vi "Configure Frequency.vi"(5 "Sweep time (ms)":dbl caption="Sweep time for zero span (ms)", 7 "Mode (Center/Span)":enum16{"Center/Span", "Start/Stop"}(ring), 8 "error in (no error)":errorcluster, 9 "Span/Stop Frequency [Hz]":dbl, 10 "Center/Start Frequency [Hz]":dbl, 11 "MXA in":refnum<class "MXA.lvclass">) -> (0 "error out":errorcluster, 3 "MXA out":refnum<class "MXA.lvclass">)   [LabVIEW 2020, in "MXA.lvclass"]
uses:
  MXA.lvclass
  C:/Sandbox/Git_Sandbox/WiSpry Test Framework source code (LV20)/WiSpry Test Framework/Instruments/Instrument.lvclass
  C:/Sandbox/Git_Sandbox/WiSpry Test Framework source code (LV20)/WiSpry Test Framework/Instruments/Spectrum Analyzer/Spectrum Analyzer.lvclass
  Instrument.lvclass/Instrument.ctl
  Spectrum Analyzer.lvclass/Spectrum Analyzer.ctl
  <instrlib>/Agilent MXA Series/Public/Configure/Configure Frequency (Start Stop).vi
  <instrlib>/Agilent MXA Series/Public/Configure/Configure Frequency (Center Span).vi
  Instrument.lvclass
  <instrlib>/Agilent MXA Series/Agilent MXA Series.lvlib
  Spectrum Analyzer.lvclass
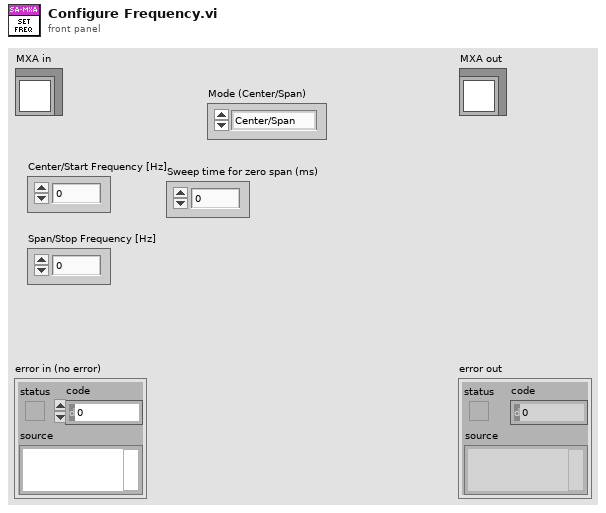
[diagram p1: front panel]
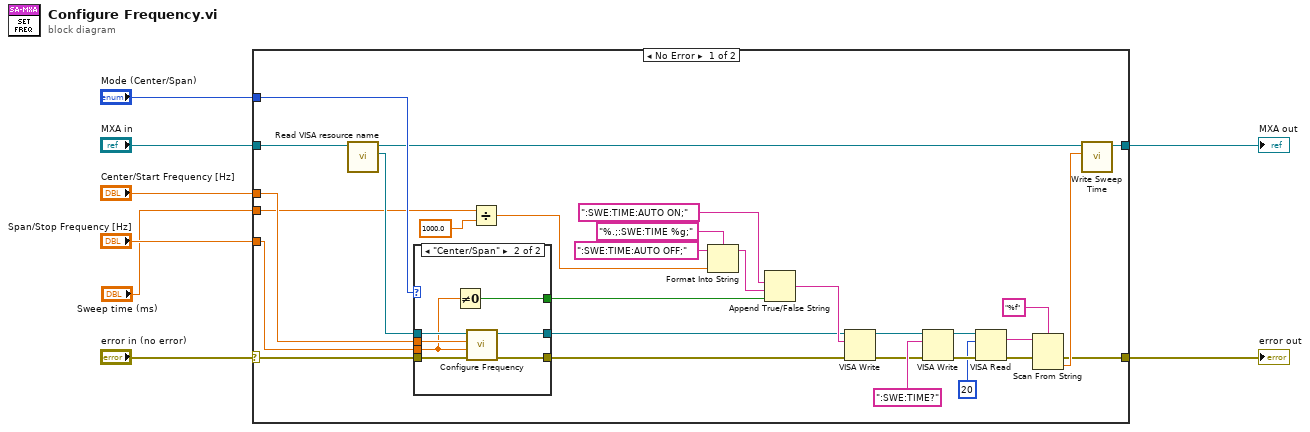
[diagram p0: block diagram]
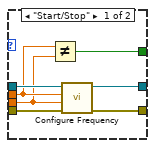
[diagram p2: hidden frame]
diagram:
  n1 = case shown="No Error" "error in (no error)" {
    selector: "error in (no error)" -> [w36 w54]
    tunnel: "MXA in" -> [w38 w53]
    tunnel: [w24 w54] -> w7
    tunnel: [w22 w53] -> w6
    tunnel: "Center/Start Frequency [Hz]" -> [w35 _]
    tunnel: "Span/Stop Frequency [Hz]" -> [w34 _]
    tunnel: "Mode (Center/Span)" -> [w33 _]
    tunnel: "Sweep time (ms)" -> [w16 _]
    frame No Error {
      n2 = call "Read VISA resource name.vi"("Instrument in"=w38) -> ("VISA resource name"=w37:refnum<visa-resource-name>, "Instrument out"=w23:refnum<class "MXA.lvclass">)  [unwired: 9 in]
      n3 = case shown="\"Center/Span\"" w33 {
        tunnel: w37 -> [w45 w52]
        tunnel: w36 -> [w44 w51]
        tunnel: [w43 w50] -> w11
        tunnel: w35 -> [w41 w49]
        tunnel: w34 -> [w40 w47]
        tunnel: [w42 w48] -> w12
        tunnel: [w39 w46] -> w17
        frame "Start/Stop" {
          n4 = Not Equal?(x=w41, y=w40) -> (x != y?=w39:bool)
          n5 = call-poly <instrlib>:"Configure Frequency.vi"("error in (no error)"=w44, "Stop Frequency (2.65E+10 Hz)"=w40, "Start Frequency (1E+7 Hz)"=w41, "VISA resource name"=w45) -> ("error out"=w43:errorcluster, "VISA resource name out"=w42:refnum<visa-resource-name>)  [unwired: 6 in]
        }
        frame "Center/Span" {
          n6 = Not Equal To 0?(x=w47) -> (x != 0?=w46:bool)
          n7 = call-poly <instrlib>:"Configure Frequency.vi"("error in (no error)"=w51, "Span (2.65E+10 Hz)"=w47, "Center Frequency (1.325E+10 Hz)"=w49, "VISA resource name"=w52) -> ("error out"=w50:errorcluster, "VISA resource name out"=w48:refnum<visa-resource-name>)  [unwired: 6 in]
        }
      }
      n8 = Divide(x=w16, y=1000.0) -> (x/y=w14:dbl)
      n9 = Format Into String(format string="%.;:SWE:TIME %g;", initial string=":SWE:TIME:AUTO OFF;", w14) -> (resulting string=w21:string)  [unwired: 1 in, 1 out]
      n10 = Append True/False String(1:w17, 2:w21, 3:":SWE:TIME:AUTO ON;") -> (0:w13:string)  [unwired: 1 in]
      n11 = VISA Write(VISA resource name=w12, write buffer=w13, error in (no error)=w11) -> (VISA resource name out=w10:refnum<visa-resource-name>, error out=w9:errorcluster)  [unwired: 1 out]
      n12 = VISA Write(VISA resource name=w10, write buffer=":SWE:TIME?", error in (no error)=w9) -> (VISA resource name out=w32:refnum<visa-resource-name>, error out=w31:errorcluster)  [unwired: 1 out]
      n13 = VISA Read(VISA resource name=w32, byte count=u32 20, error in (no error)=w31) -> (read buffer=w27:string, error out=w28:errorcluster)  [unwired: 2 out]
      n14 = Scan From String(format string="%f", input string=w27, error in=w28) -> (error out=w24:errorcluster, output 1=w25:dbl)  [unwired: 2 in, 2 out]
      n15 = call "Write Sweep Time.vi"("Sweep Time"=w25, "Spectrum Analyzer in"=w23) -> ("Spectrum Analyzer out"=w22:refnum<class "MXA.lvclass">)  [unwired: 9 in]
    }
    frame Error {
    }
  }
  "error out" <- w7
  "MXA out" <- w6
